vi "Load Project Files.vi"(0 "NI Digital in":refnum<k15>, 5 "Project Files":T1, 11 "error in (no error)":errorcluster) -> (4 "NI Digital out":refnum<k15>, 15 "error out":errorcluster)   [LabVIEW 2018, in "Digital.lvlib"]
uses:
  Digital.lvlib
  Type Definitions/Project Files.ctl
  <instrlib>/niDigital/niDigital.llb/niDigital Load Specifications Levels and Timing (Multiple).vi
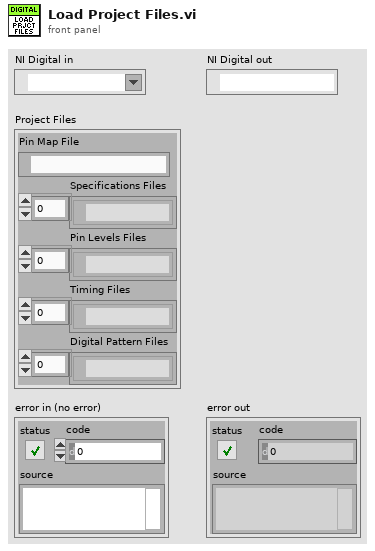
[diagram p1: front panel]
types:
  T1 = typedef "Digital.lvlib/Project Files.ctl" = cluster{"Pin Map File":path, "Specifications Files":path[], "Pin Levels Files":path[], "Timing Files":path[], "Digital Pattern Files":path[]}
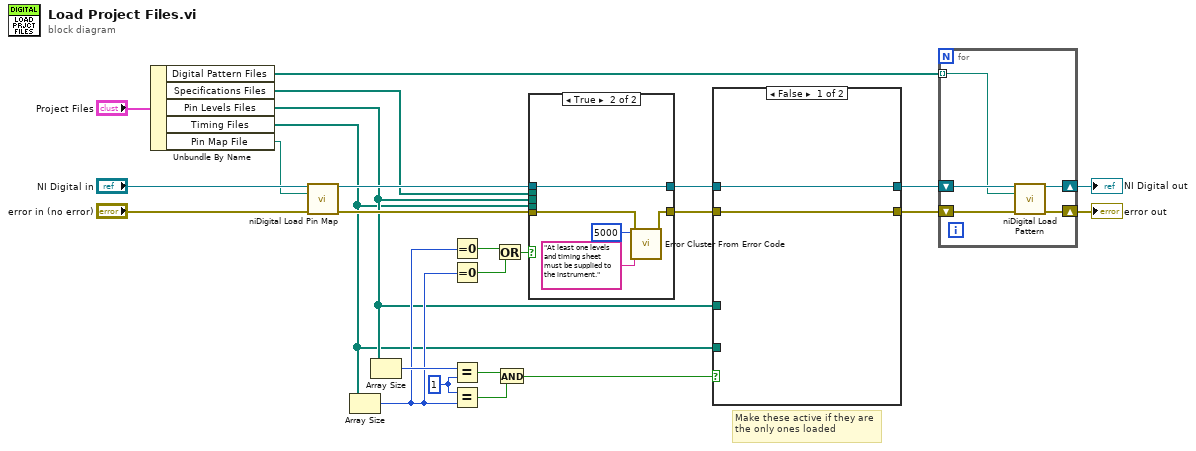
[diagram p0: block diagram]
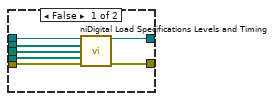
[diagram p2: hidden frame]
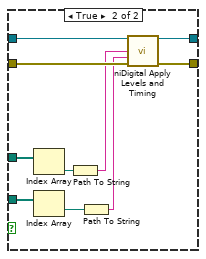
[diagram p3: hidden frame]
diagram:
  w17 = 1 ("y")
  # "Make these active if they are the only ones loaded"
  n1 = Unbundle By Name("Project Files") -> ("Digital Pattern Files"=w18:path[], "Specifications Files"=w19:path[], "Pin Levels Files"=w2:path[], "Timing Files"=w1:path[], "Pin Map File"=w21:path)
  n2 = call <instrlib>:"niDigital Load Pin Map.vi"("instrument handle"="NI Digital in", "pin map file"=w21, "error in"="error in (no error)") -> ("instrument handle out"=w20:refnum<k15>, "error out"=w23:errorcluster)  [unwired: 11 in]
  n3 = Array Size(array=w1) -> (size(s)=w12:i32)
  n4 = Array Size(array=w2) -> (size(s)=w16:i32)
  n5 = Equal To 0?(x=w12) -> (x = 0?=w11:bool)
  n6 = Equal To 0?(x=w12) -> (x = 0?=w10:bool)
  n7 = Equal?(x=w16, y=w17) -> (x = y?=w15:bool)
  n8 = Equal?(x=w17, y=w12) -> (x = y?=w14:bool)
  n9 = Or(x=w11, y=w10) -> (x .or. y?=w9:bool)
  n10 = And(x=w15, y=w14) -> (x .and. y?=w13:bool)
  n11 = case shown="True" w9 {
    tunnel: w23 -> [w32 w36]
    tunnel: [w31 w35] -> w7
    tunnel: w20 -> [w30 w37]
    tunnel: w19 -> [w29 _]
    tunnel: [w28 w37] -> w8
    tunnel: w1 -> [w27 _]
    tunnel: w2 -> [w26 _]
    frame False {
      n12 = call-poly <instrlib>:"niDigital Load Specifications Levels and Timing.vi"("instrument handle"=w30, "specifications file paths"=w29, "levels file paths"=w26, "timing file paths"=w27, "error in"=w32) -> ("instrument handle out"=w28:refnum<k15>, "error out"=w31:errorcluster)  [unwired: 9 in]
    }
    frame True {
      n13 = call <vilib>:"Error Cluster From Error Code.vi"("error in (no error)"=w36, "error message (\"\")"="At least one levels and timing sheet must be supplied to the instrument." ("error message (\"\")"), "error code (0)"=5000) -> ("error out"=w35:errorcluster)  [unwired: 6 in]
    }
  }
  n14 = case shown="False" w13 {
    tunnel: w7 -> [w38 w49]
    tunnel: [w38 w48] -> w5
    tunnel: w8 -> [w39 w47]
    tunnel: [w39 w46] -> w6
    tunnel: w2 -> [_ w42]
    tunnel: w1 -> [_ w45]
    frame False {
    }
    frame True {
      n15 = Index Array(array=w42) -> (element=w41:path)  [unwired: 1 in]
      n16 = Index Array(array=w45) -> (element=w44:path)  [unwired: 1 in]
      n17 = Path To String(path=w41) -> (string=w40:string)
      n18 = Path To String(path=w44) -> (string=w43:string)
      n19 = call <instrlib>:"niDigital Apply Levels and Timing.vi"("instrument handle"=w47, "levels sheet"=w40, "timing sheet"=w43, "error in"=w49) -> ("instrument handle out"=w46:refnum<k15>, "error out"=w48:errorcluster)  [unwired: 10 in]
    }
  }
  n20 = for {
    shift-right: [w53] -> w3
    shift-left: w5 -> [w54]
    shift-right: [w51] -> w4
    shift-left: w6 -> [w52]
    tunnel: w18 -> [w50] mode=indexing
    n21 = call <instrlib>:"niDigital Load Pattern.vi"("instrument handle"=w52, "pattern file"=w50, "error in"=w54) -> ("instrument handle out"=w51:refnum<k15>, "error out"=w53:errorcluster)  [unwired: 11 in]
  }
  "NI Digital out" <- w4
  "error out" <- w3
